vi "Set Saturation Event.vi"(8 "error in (no error)":errorcluster, 11 "saturationEvent":u32) -> (0 "error out":errorcluster, 2 "function return":u32, 3 "saturationEvent out":u32)   [LabVIEW 2014, in "atmcd32d.lvlib"]
doc: "unsigned int WINAPI SetSaturationEvent(HANDLE saturationEvent);"
uses:
  atmcd32d.lvlib
  atmcd32d.dll
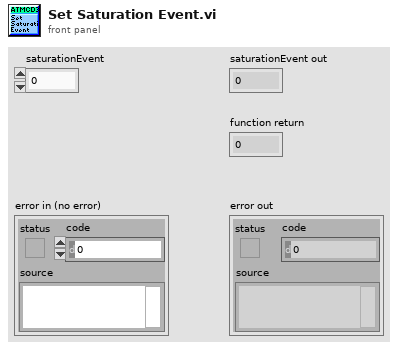
[diagram p1: front panel]
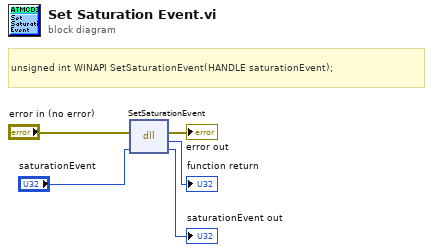
[diagram p0: block diagram]
diagram:
  # "unsigned int WINAPI SetSaturationEvent(HANDLE saturationEvent);"
  n1 = dll-call lib="C:/Users/Bakir/Documents/Lambda2-Testing/lib/Andorlib/atmcd32d.*" fn="SetSaturationEvent"(error in="error in (no error)", "saturationEvent"="saturationEvent") -> (error out=→"error out":errorcluster, →"function return":u32, "saturationEvent"=→"saturationEvent out":u32)  [unwired: 2 in, 1 out]
